vi "Get Is Turned ON.vi"(8 "error in (no error)":errorcluster, 11 "Switchable Device in":refnum<class "Switchable Device.lvclass">) -> (0 "error out":errorcluster, 2 "Is Turned ON?":bool, 3 "Switchable Device out":refnum<class "Switchable Device.lvclass">)   [LabVIEW 2018, in "Switchable Device.lvclass"]
uses:
  Switchable Device.lvclass
  Switchable Device.lvclass/Switchable Device.ctl
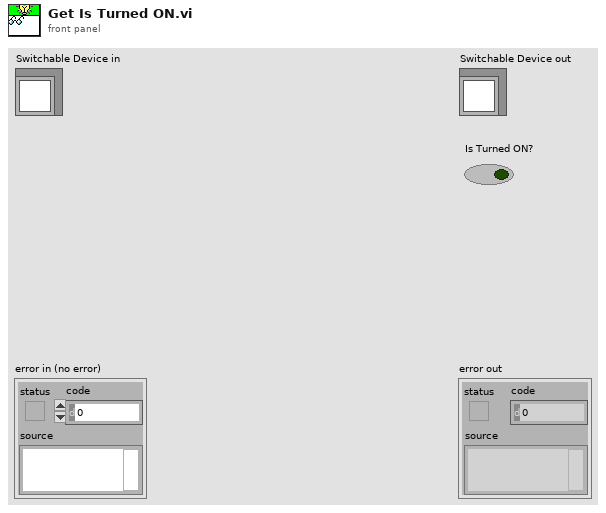
[diagram p1: front panel]
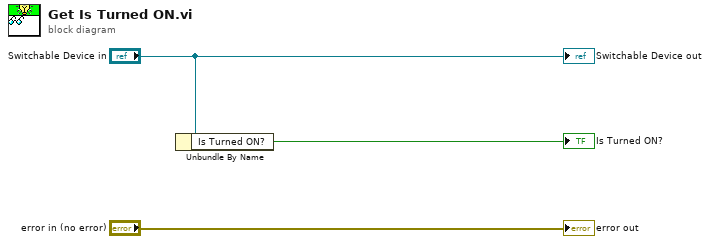
[diagram p0: block diagram]
diagram:
  n1 = Unbundle By Name("Switchable Device in") -> ("Is Turned ON?"=→"Is Turned ON?":bool)
  "error out" <- "error in (no error)"
  "Switchable Device out" <- "Switchable Device in"
